vi "ma_Check multi tone detection iteration condition.vi"(2 "precision":dbl=0.001 format="%.2e", 3 "peaks before":T1(array[cluster]) {"phase [degree]" format="%.2f"; "amplitude" format="%.2f"; "frequency [Hz]" format="%.2f"}, 4 "peaks after":T1(array[cluster]) {"phase [degree]" format="%.2f"; "amplitude" format="%.2f"; "frequency [Hz]" format="%.2f"}) -> (0 "stable?":bool[](array[boolean]), 1 "all stable?":bool)   [LabVIEW 2020, in "NI_MAPro.lvlib"]
uses:
  NI_MAPro.lvlib
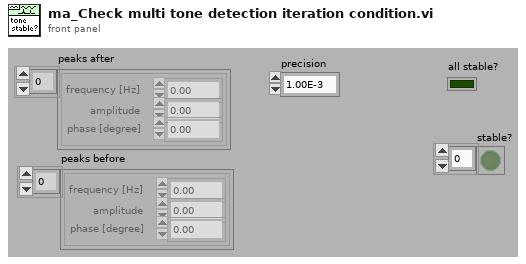
[diagram p1: front panel]
types:
  T1 = cluster{"frequency [Hz]":dbl, "amplitude":dbl, "phase [degree]":dbl}[]
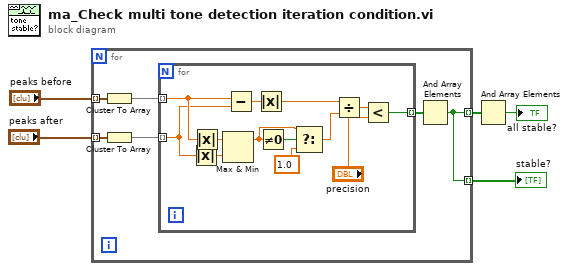
[diagram p0: block diagram]
diagram:
  n1 = for {
    tunnel: "peaks before" -> [w11] mode=indexing
    tunnel: "peaks after" -> [w10] mode=indexing
    tunnel: [w6] -> w3 mode=indexing
    tunnel: [w6] -> w1 mode=indexing
    n2 = Cluster To Array(cluster=w11) -> (array=w9:dbl[])
    n3 = Cluster To Array(cluster=w10) -> (array=w8:dbl[])
    n4 = for {
      tunnel: w9 -> [w19] mode=indexing
      tunnel: w8 -> [w18] mode=indexing
      tunnel: [w12] -> w7 mode=indexing
      n5 = Absolute Value(x=w18) -> (abs(x)=w23:dbl)
      n6 = Absolute Value(x=w19) -> (abs(x)=w24:dbl)
      n7 = Max & Min(x=w24, y=w23) -> (max(x,y)=w21:dbl)  [unwired: 1 out]
      n8 = Subtract(x=w19, y=w18) -> (x-y=w17:dbl)
      n9 = Absolute Value(x=w17) -> (abs(x)=w16:dbl)
      n10 = Not Equal To 0?(x=w21) -> (x != 0?=w22:bool)
      n11 = Select(t=w21, s=w22, f=1.0) -> (s? t:f=w15:dbl)
      n12 = Divide(x=w16, y=w15) -> (x/y=w14:dbl)
      n13 = Less?(x=w14, y="precision") -> (x < y?=w12:bool)
    }
    n14 = And Array Elements(Boolean array=w7) -> (logical AND=w6:bool)
  }
  "stable?" <- w1
  n15 = And Array Elements(Boolean array=w3) -> (logical AND=→"all stable?":bool)
